vi "Get Relay State.vi"(8 "error in (no error)":errorcluster, 10 "SLSC Switch in":refnum<class "SLSC Switch.lvclass">, 11 "RelayInterface in":refnum<class "RelayInterface.lvclass">) -> (0 "error out":errorcluster, 1 "RelayPosition":T1=10 caption="position" items=["Open"=10, "Closed"=11], 2 "SLSC Switch out":refnum<class "SLSC Switch.lvclass">, 3 "RelayInterface out":refnum<class "RelayInterface.lvclass">)   [LabVIEW 2015, in "RelayInterface.lvclass"]
uses:
  RelayInterface.lvclass
  slscsl/RelayPosition.ctl
  SLSC Switch/SLSC Switch.lvclass
  slscsl/slscsl.lvclass
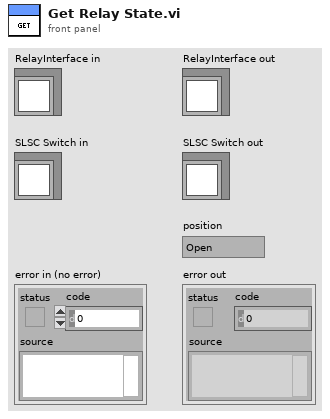
[diagram p1: front panel]
types:
  T1 = typedef "slscsl.lvclass/RelayPosition.ctl" = i32
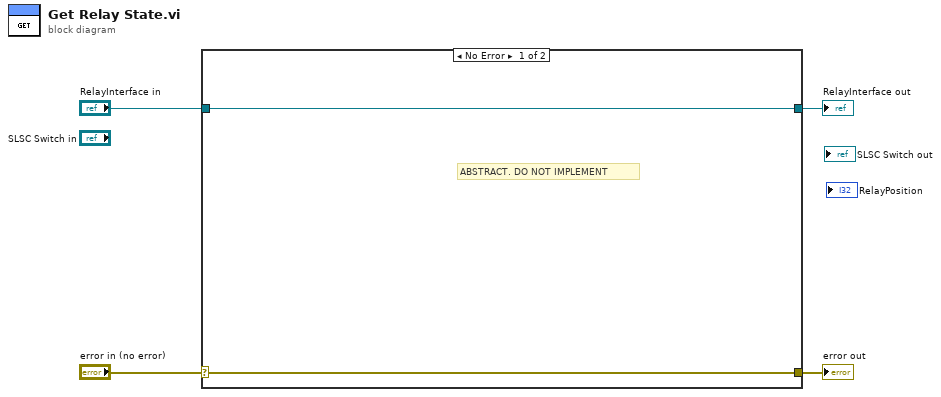
[diagram p0: block diagram]
diagram:
  n1 = case shown="No Error" "error in (no error)" {
    selector: "error in (no error)" -> [w6 w8]
    tunnel: [w6 w8] -> w3
    tunnel: [w5 w7] -> w1
    tunnel: "RelayInterface in" -> [w5 w7]
    frame No Error {
      # "ABSTRACT. DO NOT IMPLEMENT"
    }
    frame Error {
    }
  }
  "error out" <- w3
  "RelayInterface out" <- w1
